vi "P9P14_Temp_Queue_Commands.vi"(1 "P9-P14 T-Cluster -Control":T1 {"Approach" items=["Fast Settle", "No O'Shoot"]}, 3 "Queue":refnum<queue>) -> (0 "P9-P14 T-New Status":T1 {"Approach" items=["Fast Settle", "No O'Shoot"]})   [LabVIEW 2019]
uses:
  PPMS/P9P14-TCluster-Control.ctl
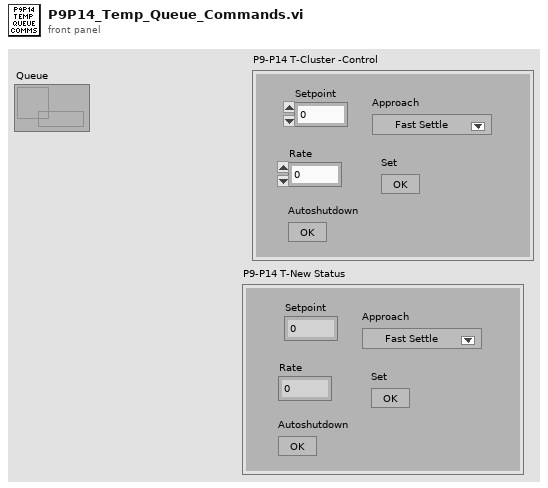
[diagram p1: front panel]
types:
  T1 = typedef "P9P14-TCluster-Control.ctl" = cluster{"Setpoint":dbl, "Rate":dbl, "Approach":u16, "Set":bool, "Autoshutdown":bool}
  T2 = cluster{"Setpoint":bool, "Rate":bool, "Approach":bool, "Set":bool, "Autoshutdown":bool}
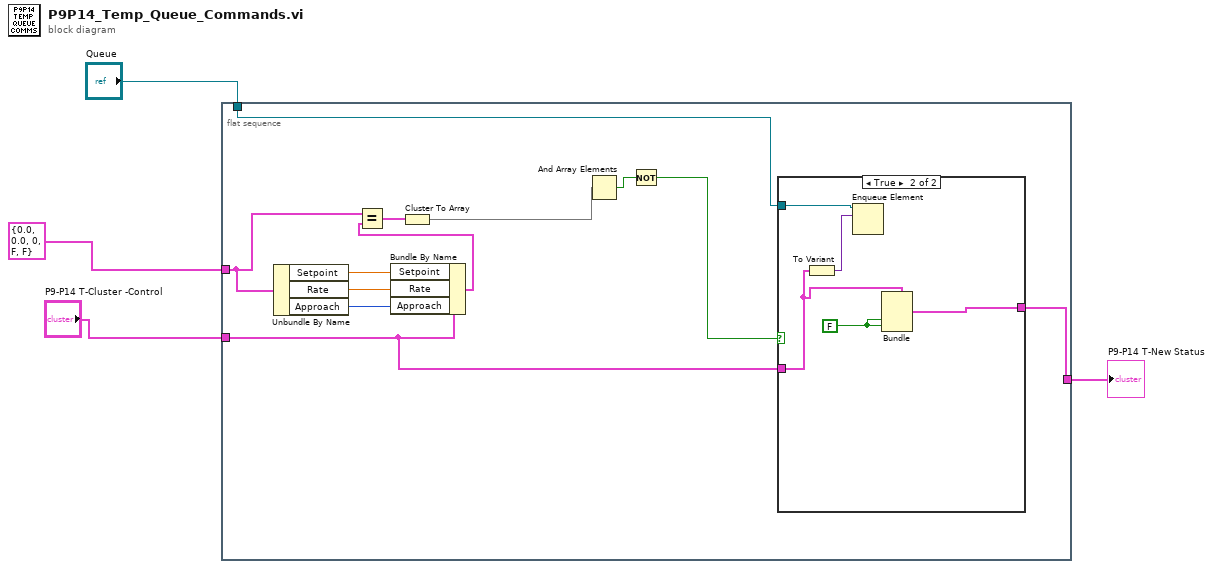
[diagram p0: block diagram]
diagram:
  n1 = flat-sequence {
    tunnel: "Queue" -> [w6]
    tunnel: T1 {"Setpoint"=0.0, "Rate"=0.0, "Approach"=0, "Set"=FALSE, "Autoshutdown"=FALSE} ("P9-P14 T-Last Status") -> [w13]
    tunnel: "P9-P14 T-Cluster -Control" -> [w7]
    tunnel: [w5] -> w1
    frame #0 {
      n2 = Unbundle By Name(w13) -> ("Setpoint"=w16:dbl, "Rate"=w15:dbl, "Approach"=w14:u16)
      n3 = Bundle By Name(cluster=w7, "Setpoint"=w16, "Rate"=w15, "Approach"=w14) -> (w12:T1)
      n4 = Equal?(x=w13, y=w12) -> (x = y?=w9:T2)
      n5 = Cluster To Array(cluster=w9) -> (array=w11:bool[])
      n6 = And Array Elements(Boolean array=w11) -> (logical AND=w10:bool)
      n7 = Not(x=w10) -> (.not. x?=w8:bool)
      n8 = case shown="True" w8 {
        tunnel: w7 -> [w17 w20]
        tunnel: w6 -> [_ w22]
        tunnel: [w17 w19] -> w5
        frame False {
        }
        frame True {
          w18 = FALSE
          n9 = To Variant(anything=w20) -> (Variant=w21:variant)
          n10 = Enqueue Element(queue=w22, element=w21) -> ()  [unwired: 2 in, 3 out]
          n11 = Bundle(cluster=w20, "Set"=w18, "Autoshutdown"=w18) -> (w19:T1)  [unwired: 3 in]
        }
      }
    }
  }
  "P9-P14 T-New Status" <- w1
